vi "Actor Core.vi"(8 "error in":errorcluster, 11 "Right Panel in":refnum<class "Debugger.lvclass">) -> (0 "error out":errorcluster, 3 "Actor out":refnum<class "Actor.lvclass">)   [LabVIEW 2023, in "Debugger.lvlib" / "Debugger.lvclass"]
doc: "Base Class for the right subpanel.\nThis provides the basic implementation for show/hide operations.\n\nancestor classes should override this, but maintain proportions."
uses:
  Library/Debugger.lvclass
  builds/Framework/Actor Framework.lvlibp/1abvi3w/vi.lib/ActorFramework/Actor/Actor.lvclass
  builds/Main/Docking.lvlibp/Right Panel/RightDock.lvclass
  builds/Framework/Engine.lvlibp/Engine/Library/Engine.lvclass
panel:
  in  "GenerateError":bool
  in  "GenerateWarning":bool
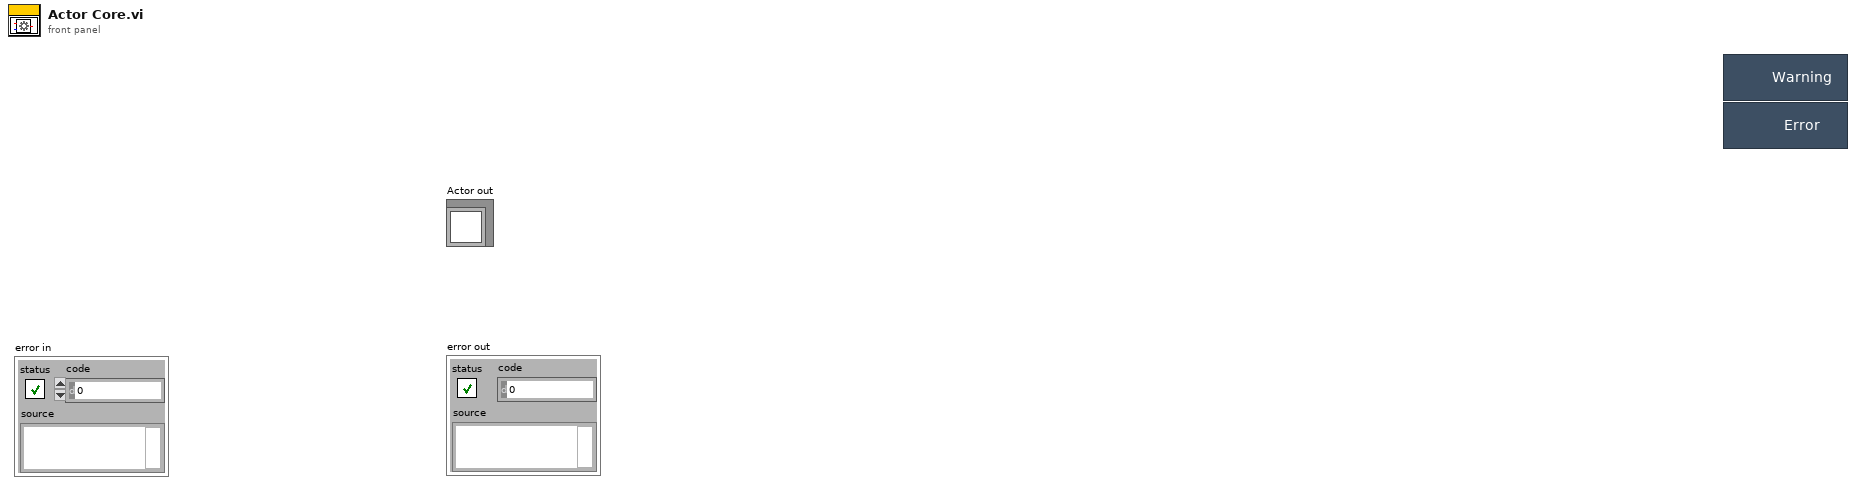
[diagram p1: front panel]
types:
  T1 = cluster{"Pnl Actor":refnum<event-registration>, "Event Registration Refnum":refnum<event-registration>}
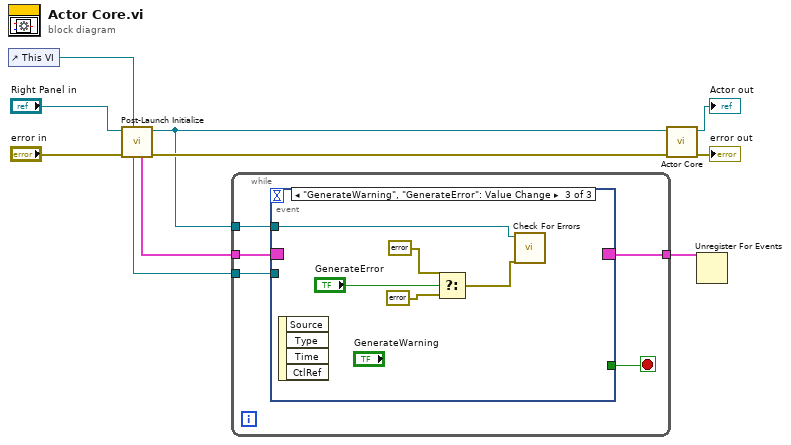
[diagram p0: block diagram]
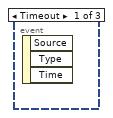
[diagram p2: hidden frame]
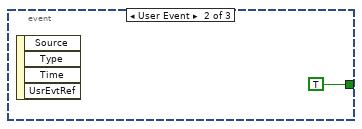
[diagram p3: hidden frame]
diagram:
  n1 = control-ref of="This VI"() -> (w1:refnum<vi>)
  n2 = call "Post-Launch Initialize.vi"("GUI Reference"=w1, "error in (no error)"="error in", "Engine in"="Right Panel in") -> ("error out"=w7:errorcluster, "Engine out"=w2:refnum<class "Debugger.lvclass">, "Registered Events"=w4:T1, "Self Enqueuer"=w3:refnum<class "Message Enqueuer.lvclass">)  [unwired: 5 in]
  n3 = while {
    tunnel: [w15] -> w5
    tunnel: w4 -> [w14]
    tunnel: w3 -> [w13]
    tunnel: w2 -> [w11]
    stop <- w12 stop-if-true
    n4 = event shown="[2] \"GenerateWarning\", \"GenerateError\": Value Change" {
      selector: w14 -> [_ _ _]
      dyn-events: [_ _ _] -> w15
      timeout: _ -> [_ _ _]
      tunnel: w13 -> [_ _ _]
      tunnel: [_ TRUE _] -> w12
      tunnel: w11 -> [_ _ w21]
      event Timeout {
        n5 = event-data() -> ()  [unwired: 1 in, 3 out]
      }
      event User Event {
        n6 = event-data() -> ()  [unwired: 1 in, 4 out]
      }
      event "GenerateWarning", "GenerateError": Value Change {
        n7 = event-data() -> ()  [unwired: 1 in, 4 out]
        n8 = Select(t=errorcluster {"status"=TRUE, "code"=-8999, "source"="Error Message"} ("error in"), s="GenerateError", f=errorcluster {"status"=FALSE, "code"=-8999, "source"="Warning Message"} ("error in")) -> (s? t:f=w18:errorcluster)
        n9 = call "Check For Errors.vi"("error in"=w18, "Engine in"=w21) -> ()  [unwired: 8 in, 2 out]
      }
    }
  }
  n10 = call-parent "Actor Core.vi"("error in"=w7, "Right Panel in"=w2) -> ("error out"=→"error out":errorcluster, "Actor out"=→"Actor out":refnum<class "Actor.lvclass">)  [unwired: 8 in]
  n11 = Unregister For Events(event registration refnum=w5) -> ()  [unwired: 1 in, 1 out]
